vi "LodFile---.vi"(8 "error in (no error)":errorcluster caption="错误输入（无错误）") -> (0 "error out":errorcluster caption="错误输出")   [LabVIEW 2018]
panel:
  out "字符串":string
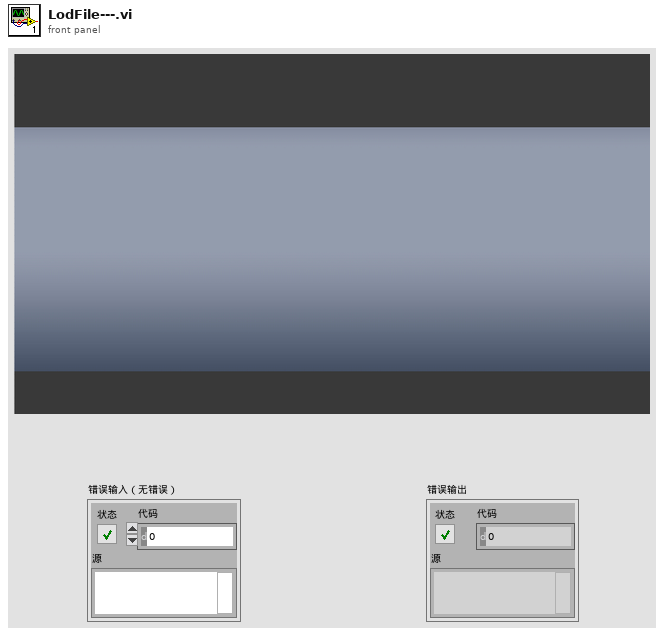
[diagram p1: front panel]
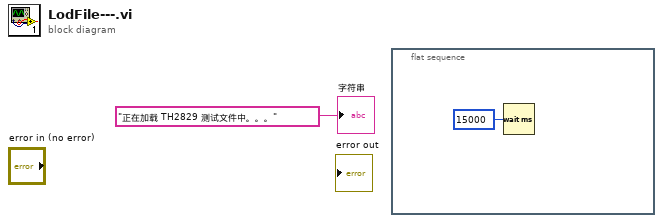
[diagram p0: block diagram]
diagram:
  n1 = flat-sequence {
    frame #0 {
      n2 = Wait (ms)(milliseconds to wait=u32 15000 ("等待时间（毫秒）")) -> ()  [unwired: 1 out]
    }
  }
  "字符串" <- "正在加载 TH2829 测试文件中。。。" ("字符串")
